vi "R And Z Register Values.vi"(8 "error in (no error)":errorcluster, 10 "Value Number (1)":i32=1 min=0 max=99, 11 "VISA resource name":refnum<visa-resource-name>) -> (0 "error out":errorcluster, 1 "Z":dbl format="%^.3e", 2 "Rn":dbl format="%^.3e", 3 "VISA resource name out":refnum<visa-resource-name>)   [LabVIEW 2010, in "Agilent 4194.lvlib"]
doc: "This function outputs the instrument's single value register data."
uses:
  <instrlib>/Agilent 4194/Agilent 4194.lvlib
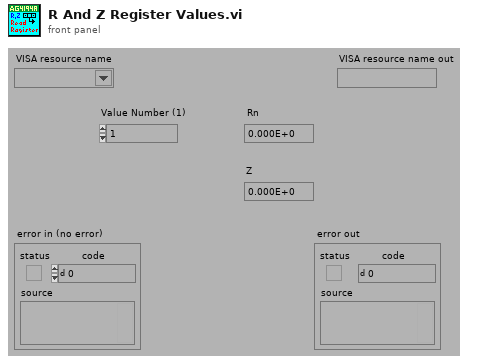
[diagram p1: front panel]
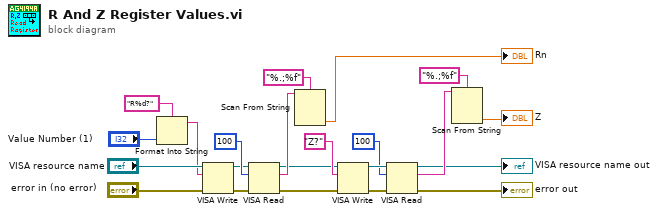
[diagram p0: block diagram]
diagram:
  n1 = Format Into String(format string="R%d?", "Value Number (1)") -> (resulting string=w6:string)  [unwired: 2 in, 1 out]
  n2 = VISA Write(VISA resource name="VISA resource name", write buffer=w6, error in (no error)="error in (no error)") -> (VISA resource name out=w18:refnum<visa-resource-name>, error out=w17:errorcluster)  [unwired: 1 out]
  n3 = VISA Read(VISA resource name=w18, byte count=u32 100 ("byte count (0)"), error in (no error)=w17) -> (VISA resource name out=w11:refnum<visa-resource-name>, read buffer=w20:string, error out=w10:errorcluster)  [unwired: 1 out]
  n4 = Scan From String(format string="%.;%f", input string=w20) -> (output 1=→"Rn":dbl)  [unwired: 3 in, 3 out]
  n5 = VISA Write(VISA resource name=w11, write buffer="Z?" ("write buffer (\"\")"), error in (no error)=w10) -> (VISA resource name out=w15:refnum<visa-resource-name>, error out=w16:errorcluster)  [unwired: 1 out]
  n6 = VISA Read(VISA resource name=w15, byte count=u32 100 ("byte count (0)"), error in (no error)=w16) -> (VISA resource name out=→"VISA resource name out":refnum<visa-resource-name>, read buffer=w13:string, error out=→"error out":errorcluster)  [unwired: 1 out]
  n7 = Scan From String(format string="%.;%f", input string=w13) -> (output 1=→"Z":dbl)  [unwired: 3 in, 3 out]
